vi "GetMemberName.vi"(8 "error in (no error)":errorcluster, 11 "ArrayElementScripter in":refnum<class "ArrayElementScripter.lvclass">) -> (0 "error out":errorcluster, 2 "MemberName":string, 3 "ArrayElementScripter out":refnum<class "ArrayElementScripter.lvclass">)   [LabVIEW 2021, in "MemberVICreation.lvlib" / "ArrayElementScripter.lvclass"]
uses:
  <resource>/Framework/Providers/LVClassLibrary/NewAccessors/ArrayElementScripter/ArrayElementScripter.lvclass
  <resource>/Framework/Providers/LVClassLibrary/NewAccessors/CLSUIP_LocalizedStrings.vi
  <resource>/Framework/Providers/LVClassLibrary/NewAccessors/MemberVICreation.lvlib
  <resource>/Framework/Providers/LVClassLibrary/NewAccessors/BaseAccessorScripter/BaseAccessorScripter.lvclass
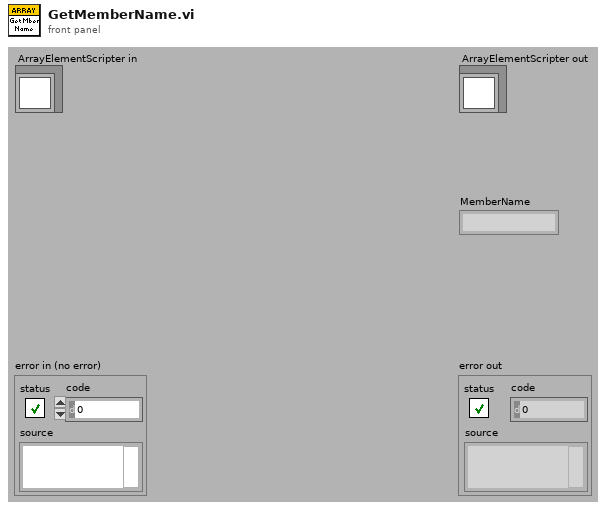
[diagram p1: front panel]
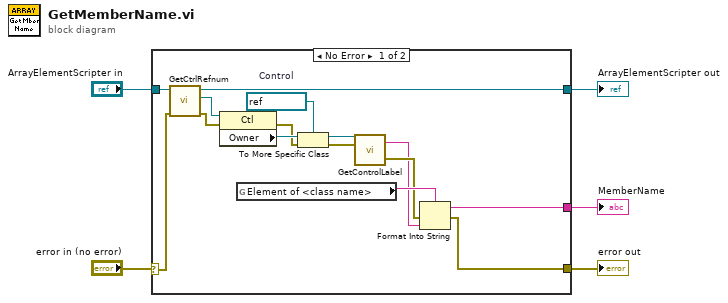
[diagram p0: block diagram]
diagram:
  n1 = case shown="No Error" "error in (no error)" {
    selector: "error in (no error)" -> [w16 w21]
    tunnel: "ArrayElementScripter in" -> [w20 w22]
    tunnel: [w19 w22] -> w3
    tunnel: [w10 _] -> w2
    tunnel: [w9 w21] -> w1
    frame No Error {
      w14 = refnum<vi> refnum  # Control
      n2 = call-dynamic "GetCtrlRefnum.vi"("error in (no error)"=w16, "BaseAccessorScripter in"=w20) -> ("error out"=w18:errorcluster, "Ctl Refnum"=w17:refnum<vi>, "BaseAccessorScripter out"=w19:refnum<class "ArrayElementScripter.lvclass">)  [unwired: 7 out]
      n3 = property class="Ctl"(reference=w17, error in=w18) -> (error out=w13:errorcluster, "Owner"=w15:refnum<vi>)  [unwired: 1 out]
      n4 = global read "CLSUIP_LocalizedStrings.vi" "Element of <class name>"() -> (w8:string)
      n5 = To More Specific Class(target class=w14, reference=w15, error in=w13) -> (specific class reference=w12:refnum<vi>, error out=w11:errorcluster)
      n6 = call <resource>:"GetControlLabel.vi"("error IO"=w11, "Ctl Refnum"=w12) -> ("error out"=w7:errorcluster, "Label.Text"=w6:string)
      n7 = Format Into String(format string=w8, error in=w7, w6) -> (resulting string=w10:string, error out=w9:errorcluster)  [unwired: 1 in]
    }
    frame Error {
    }
  }
  "error out" <- w1
  "MemberName" <- w2
  "ArrayElementScripter out" <- w3
